vi "Write_to_OPC_UA.vi"() -> ()   [LabVIEW 2021]
uses:
  <vilib>/OPCUA/controls/NodeId.ctl
  <vilib>/OPCUA/controls/Write Status.ctl
  <vilib>/OPCUA/client/Multiple Write Double.vi
  <vilib>/OPCUA/NI OPC UA Client.lvlib
panel:
  out "Numeric 2":dbl
  in  "Node_Id":string
  in  "server endpoint URL":string
  in  "stop":bool
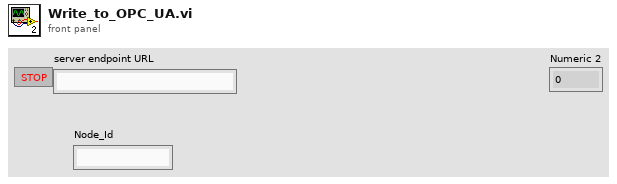
[diagram p1: front panel]
types:
  T1 = cluster{"message mode":enum16{"None", "Sign", "Sign and Encrypt"}, "security":enum16{"Basic256", "Basic128Rsa15"}}
  T2 = typedef "OPC UA Client Refnum.ctl" = refnum<k21>
  T3 = typedef "NodeId.ctl" = string
  T4 = typedef "Write Status.ctl" = u32
  T5 = cluster{"node ID":T3, "value":dbl, "timestamp (current time)":timestamp, "node status":T4}
  T6 = cluster{"node ID":T3, "value":dbl, "timestamp (current time)":timestamp, "node status":T4}[]
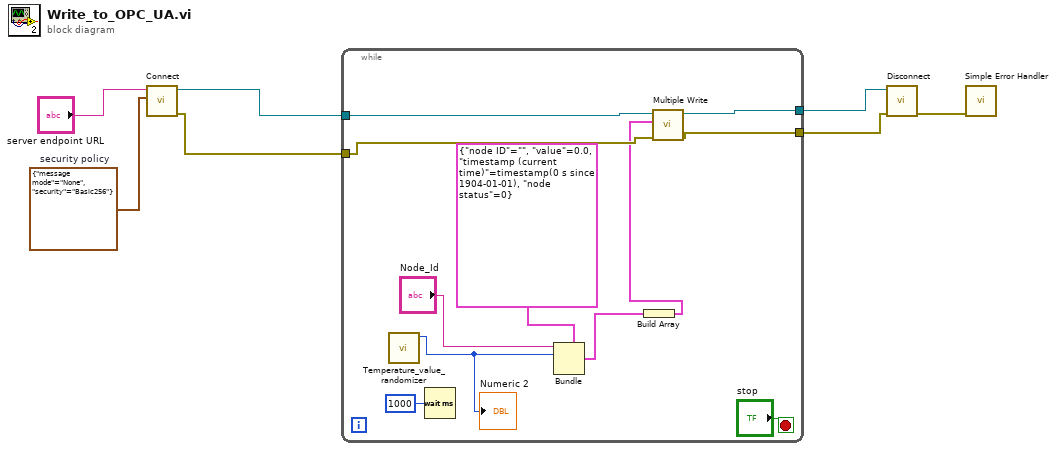
[diagram p0: block diagram]
diagram:
  w7 = T1 {"message mode"=enum."None", "security"=enum."Basic256"}  # security policy
  n1 = call <vilib>:"Connect.vi"("security policy"=w7, "server endpoint URL"="server endpoint URL") -> ("error out"=w4:errorcluster, "OPC UA client refnum out"=w5:T2)  [unwired: 7 in, 1 out]
  n2 = while {
    tunnel: w5 -> [w17]
    tunnel: w4 -> [w16]
    tunnel: [w15] -> w1
    tunnel: [w14] -> w2
    stop <- "stop" stop-if-true
    n3 = call "Temperature_value_randomizer.vi"() -> ("Temperature Value"=w10:i32)  [unwired: 11 in]
    "Numeric 2" <- w10
    n4 = Wait (ms)(milliseconds to wait=u32 1000) -> ()  [unwired: 1 out]
    n5 = Bundle(cluster=T5 {"node ID"="", "value"=0.0, "timestamp (current time)"=timestamp(0 s since 1904-01-01), "node status"=0} ("request"), "node ID"="Node_Id", "value"=w10) -> (w12:T5)  [unwired: 2 in]
    n6 = Build Array(w12) -> (w8:T6)
    n7 = call-poly <vilib>:"Multiple Write.vi"("error in (no error)"=w16, "requests"=w8, "OPC UA client refnum in"=w17) -> ("error out"=w15:errorcluster, "OPC UA client refnum out"=w14:T2)  [unwired: 5 in, 2 out]
  }
  n8 = call <vilib>:"Disconnect.vi"("error in (no error)"=w1, "OPC UA client refnum in"=w2) -> ("error out"=w3:errorcluster)  [unwired: 9 in]
  n9 = call <vilib>:"Simple Error Handler.vi"("error in (no error)"=w3) -> ()  [unwired: 4 in, 5 out]
